vi "Pointer_Delete.vi"(8 "Error":errorcluster, 9 "Name":string, 10 "Index":i32=-1, 11 "WavBuf":refnum<class "WavBuf.lvclass">) -> (0 "Error Out":errorcluster, 1 "Pointer Cluster Out":refnum<class "_Pointer.lvclass">, 2 "Index Out":i32, 3 "WavBuf Out":refnum<class "WavBuf.lvclass">, 4 "Found Out":bool)   [LabVIEW 2025, in "WavBuf.lvclass"]
uses:
  WavBuf.lvclass
  Pointer/_Pointer.lvclass
  WavBuf.lvclass/WavBuf.ctl
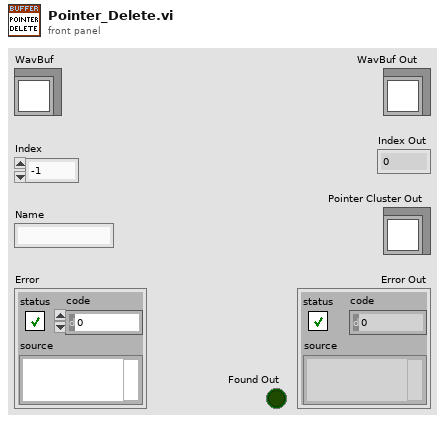
[diagram p1: front panel]
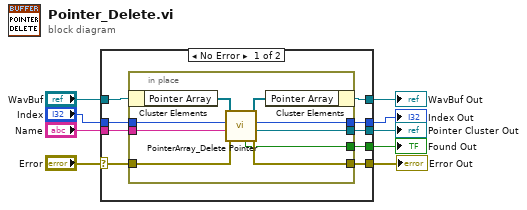
[diagram p0: block diagram]
diagram:
  n1 = case shown="No Error" "Error" {
    selector: "Error" -> [w12 w29]
    tunnel: [w11 w29] -> w8
    tunnel: [w17 w28] -> w6
    tunnel: "WavBuf" -> [w18 w28]
    tunnel: "Name" -> [w16 _]
    tunnel: "Index" -> [w15 _]
    tunnel: [w14 _] -> w3
    tunnel: [w13 _] -> w2
    tunnel: [w10 _] -> w1
    frame No Error {
      n2 = in-place {
        in-place-border: w16 -> [w26]
        in-place-border: w15 -> [w25]
        in-place-border: [w23] -> w14
        in-place-border: [w22] -> w13
        in-place-border: w12 -> [w21]
        in-place-border: [w20] -> w11
        in-place-border: [w19] -> w10
        n3 = in-place-cluster #1(w18) -> ("Pointer Array"=w27:refnum<class "_Pointer.lvclass">[])
        n4 = call "PointerArray_Delete Pointer.vi"("Error"=w21, "Name"=w26, "Index"=w25, "Pointer Array"=w27) -> ("Error Out"=w20:errorcluster, "Pointer Out"=w23:refnum<class "_Pointer.lvclass">, "Index Out"=w22:i32, "Pointer Array Out"=w24:refnum<class "_Pointer.lvclass">[], "Found Out"=w19:bool)  [unwired: 3 in]
        n5 = in-place-cluster #1("Pointer Array"=w24) -> (w17:refnum<class "WavBuf.lvclass">)
      }
    }
    frame Error {
    }
  }
  "Error Out" <- w8
  "WavBuf Out" <- w6
  "Pointer Cluster Out" <- w3
  "Index Out" <- w2
  "Found Out" <- w1
